vi "Build All.vi"(8 "Error In":errorcluster) -> (0 "Error Out":errorcluster)   [LabVIEW 2017]
panel:
  out "Tools Menu":bool
  out "Toolkit VIs":bool
  out "Shortcut Menu":bool
  out "Quick Drop":bool
  out "Bookmark Manager":bool
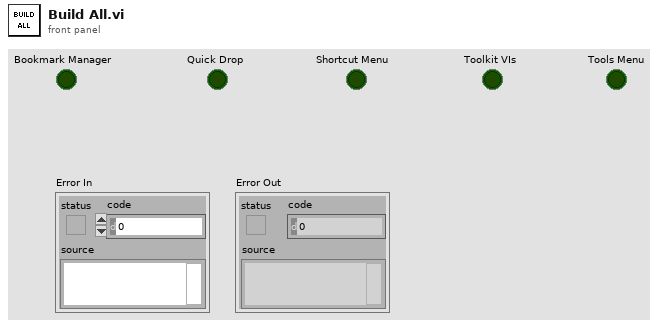
[diagram p1: front panel]
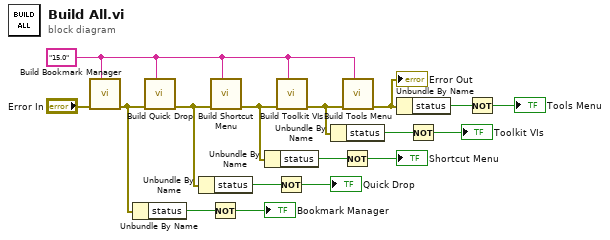
[diagram p0: block diagram]
diagram:
  w17 = "15.0" ("Target Version")
  n1 = call "Build Bookmark Manager.vi"("Target Version"=w17, "Error In"="Error In") -> ("Error Out"=w15:errorcluster)  [unwired: 9 in]
  n2 = Unbundle By Name(w15) -> ("status"=w14:bool)
  n3 = call "Build Quick Drop.vi"("Target Version"=w17, "Error In"=w15) -> ("Error Out"=w12:errorcluster)  [unwired: 9 in]
  n4 = Unbundle By Name(w12) -> ("status"=w11:bool)
  n5 = Not(x=w14) -> (.not. x?=→"Bookmark Manager":bool)
  n6 = call "Build Shortcut Menu.vi"("Target Version"=w17, "Error In"=w12) -> ("Error Out"=w6:errorcluster)  [unwired: 9 in]
  n7 = Unbundle By Name(w6) -> ("status"=w7:bool)
  n8 = Not(x=w11) -> (.not. x?=→"Quick Drop":bool)
  n9 = call "Build Toolkit VIs.vi"("Target Version"=w17, "Error In"=w6) -> ("Error Out"=w5:errorcluster)  [unwired: 9 in]
  n10 = Unbundle By Name(w5) -> ("status"=w8:bool)
  n11 = Not(x=w7) -> (.not. x?=→"Shortcut Menu":bool)
  n12 = call "Build Tools Menu.vi"("Target Version"=w17, "Error In"=w5) -> ("Error Out"=w4:errorcluster)  [unwired: 9 in]
  "Error Out" <- w4
  n13 = Unbundle By Name(w4) -> ("status"=w9:bool)
  n14 = Not(x=w8) -> (.not. x?=→"Toolkit VIs":bool)
  n15 = Not(x=w9) -> (.not. x?=→"Tools Menu":bool)
